vi "超标留样启动流程.vi"   [LabVIEW 2016, in "德润DR803L超标留样.lvlib"]
types:
  T1 = enum16{"open", "read", "write", "write single", "close"}
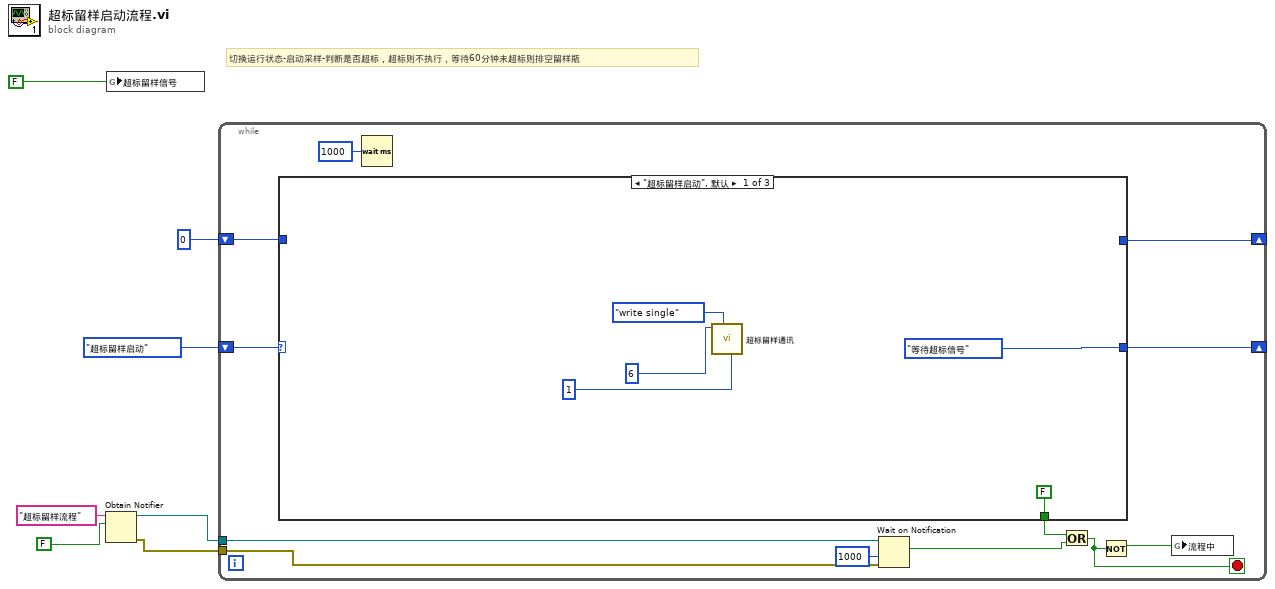
[diagram p0: block diagram]
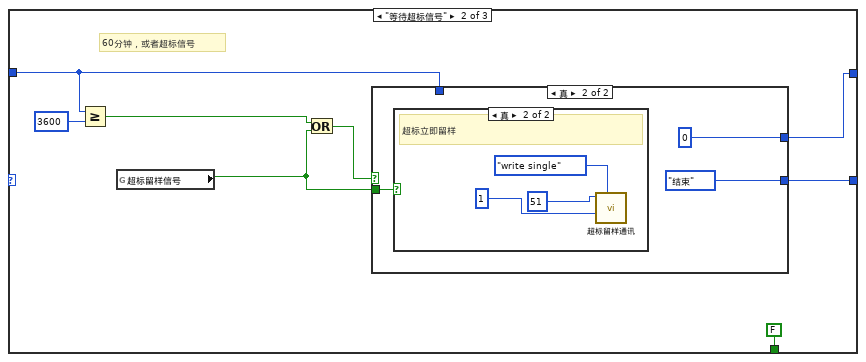
[diagram p2: hidden frame]
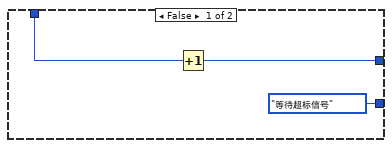
[diagram p3: hidden frame]
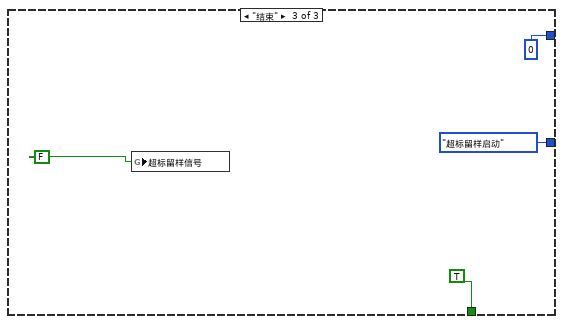
[diagram p5: hidden frame]
diagram:
  # "切换运行状态-启动采样-判断是否超标，超标则不执行，等待60分钟未超标则排空留样瓶"
  n1 = Obtain Notifier(name (unnamed)="超标留样流程" ("名称（未命名）"), notification data type=FALSE ("采样完成")) -> (notifier out=w3:refnum<notifier>, error out=w2:errorcluster)  [unwired: 2 in, 1 out]
  n2 = global write "串口参数断电保存全局变量.vi" "超标留样信号"(FALSE ("采样完成")) -> ()
  n3 = while {
    shift-right: [w10] -> _
    shift-left: enum16{"超标留样启动", "等待超标信号", "结束"}."超标留样启动" -> [w19]
    shift-right: [w16] -> _
    shift-left: 0 -> [w17]
    tunnel: w3 -> [w15]
    tunnel: w2 -> [w14]
    stop <- w12 stop-if-true
    n4 = case shown="\"超标留样启动\", 默认" w19 {
      tunnel: w17 -> [_ w28 _]
      tunnel: [_ w30 0] -> w16
      tunnel: [enum16{"超标留样启动", "等待超标信号", "结束"}."等待超标信号" w27 enum16{"超标留样启动", "等待超标信号", "结束"}."超标留样启动"] -> w10
      tunnel: [FALSE FALSE TRUE] -> w9
      frame "超标留样启动", Default {
        n5 = call "超标留样通讯.vi"("value"=u16 1 ("新元素/子数组"), "STEP"=T1."write single", "starting address"=6 ("索引")) -> ()  [unwired: 6 in, 3 out]
      }
      frame "等待超标信号" {
        # "60分钟，或者超标信号"
        n6 = Greater Or Equal?(x=w28, y=3600) -> (x >= y?=w31:bool)
        n7 = global read "串口参数断电保存全局变量.vi" "超标留样信号"() -> (w25:bool)
        n8 = Or(x=w31, y=w25) -> (x .or. y?=w29:bool)
        n9 = case shown="真" w29 {
          tunnel: [enum16{"超标留样启动", "等待超标信号", "结束"}."等待超标信号" enum16{"超标留样启动", "等待超标信号", "结束"}."结束"] -> w27
          tunnel: w28 -> [w35 _]
          tunnel: [w34 0] -> w30
          tunnel: w25 -> [_ w36]
          frame False {
            n10 = Increment(x=w35) -> (x+1=w34:i32)
          }
          frame True {
            n11 = case shown="真" w36 {
              frame False {
              }
              frame True {
                # "超标立即留样"
                n12 = call "超标留样通讯.vi"("value"=u16 1 ("新元素/子数组"), "STEP"=T1."write single", "starting address"=51 ("索引")) -> ()  [unwired: 6 in, 3 out]
              }
            }
          }
        }
      }
      frame "结束" {
        n13 = global write "串口参数断电保存全局变量.vi" "超标留样信号"(FALSE ("采样完成")) -> ()
      }
    }
    n14 = Wait (ms)(milliseconds to wait=u32 1000 ("等待时间（毫秒）")) -> ()  [unwired: 1 out]
    n15 = Wait on Notification(notifier=w15, timeout in ms (-1)=1000 ("超时毫秒(-1)"), error in (no error)=w14) -> (notification=w11:bool)  [unwired: 1 in, 3 out]
    n16 = Or(x=w9, y=w11) -> (x .or. y?=w12:bool)
    n17 = Not(x=w12) -> (.not. x?=w8:bool)
    n18 = global write "串口参数断电保存全局变量.vi" "流程中"(w8) -> ()
  }
